vi "Get Active Row.vi"(8 "error in (no error)":errorcluster, 11 "Loop Data":T1) -> (0 "error out":errorcluster, 3 "Loop Data out":T1)   [LabVIEW 2016, in "System Mapping Tool.lvlib"]
uses:
  System Mapping Tool.lvlib
  TypeDefs/Loop Data.ctl
  TypeDefs/UI Refs.ctl
  NationalInstruments.VeriStand.SystemDefinitionAPI
  NationalInstruments.VeriStand.SystemStorageUI
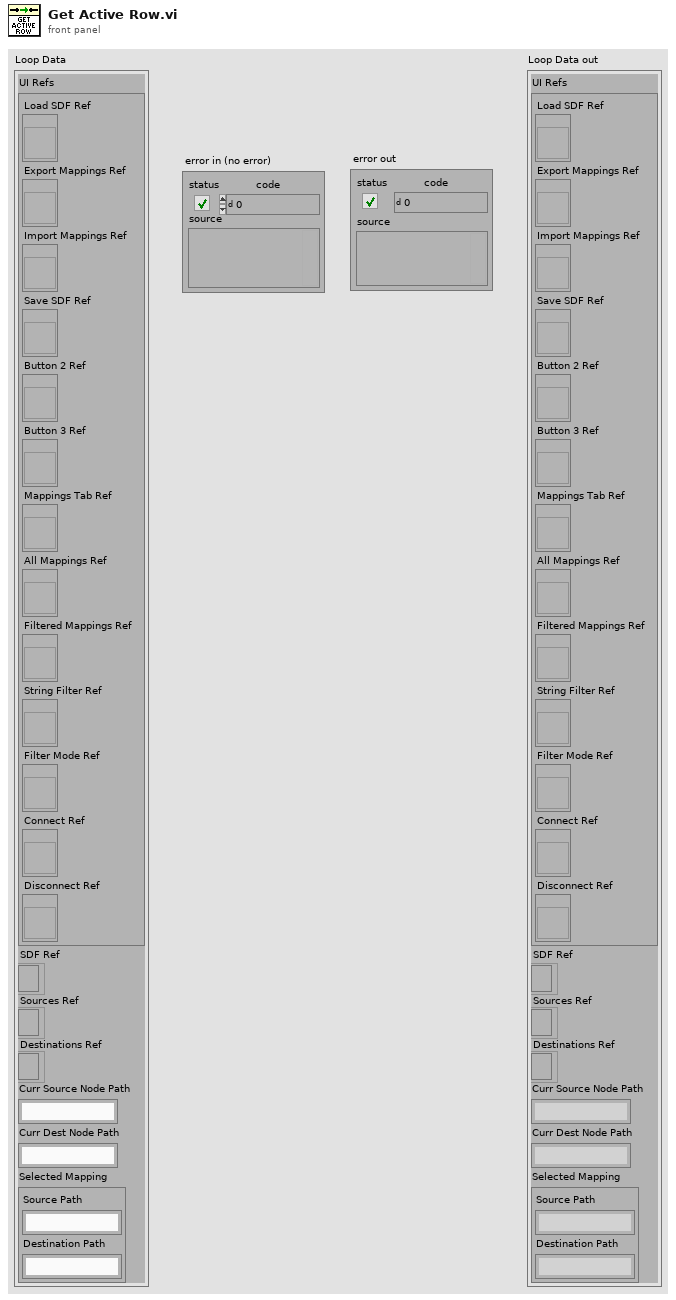
[diagram p1: front panel]
types:
  T1 = typedef "System Mapping Tool.lvlib/Loop Data.ctl" = cluster{"UI Refs":T2, "SDF Ref":refnum<k24>, "Sources Ref":refnum<k24>, "Destinations Ref":refnum<k24>, "Curr Source Node Path":string, "Curr Dest Node Path":string, "Selected Mapping":cluster{"Source Path":string, "Destination Path":string}}
  T2 = typedef "System Mapping Tool.lvlib/UI Refs.ctl" = cluster{"Load SDF Ref":refnum<vi>, "Export Mappings Ref":refnum<vi>, "Import Mappings Ref":refnum<vi>, "Save SDF Ref":refnum<vi>, "Button 2 Ref":refnum<vi>, "Button 3 Ref":refnum<vi>, "Mappings Tab Ref":refnum<vi>, "All Mappings Ref":refnum<vi>, "Filtered Mappings Ref":refnum<vi>, "String Filter Ref":refnum<vi>, "Filter Mode Ref":refnum<vi>, "Connect Ref":refnum<vi>, "Disconnect Ref":refnum<vi>}
  T3 = enum32{"All System Mappings", "Filtered Mappings by Node"}
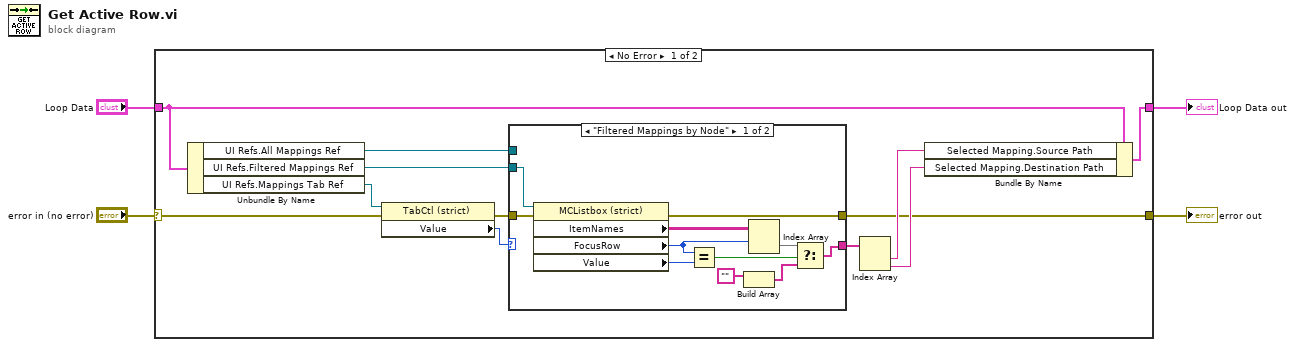
[diagram p0: block diagram]
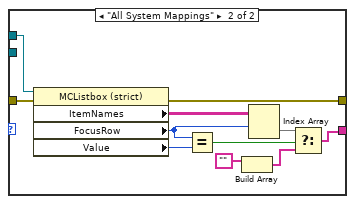
[diagram p2: hidden frame]
diagram:
  n1 = case shown="No Error" "error in (no error)" {
    selector: "error in (no error)" -> [w14 w40]
    tunnel: [w5 w40] -> w3
    tunnel: "Loop Data" -> [w16 w39]
    tunnel: [w15 w39] -> w1
    frame No Error {
      n2 = Unbundle By Name(w16) -> ("UI Refs.All Mappings Ref"=w9:refnum<vi>, "UI Refs.Filtered Mappings Ref"=w10:refnum<vi>, "UI Refs.Mappings Tab Ref"=w13:refnum<vi>)
      n3 = property class="TabCtl (strict)"(reference=w13, error in=w14) -> (error out=w11:errorcluster, "Value"=w12:T3)  [unwired: 1 out]
      n4 = case shown="\"Filtered Mappings by Node\"" w12 {
        tunnel: w11 -> [w27 w38]
        tunnel: w10 -> [w26 _]
        tunnel: w9 -> [_ w35]
        tunnel: [w24 w36] -> w5
        tunnel: [w19 w32] -> w8
        frame "Filtered Mappings by Node" {
          w22 = ""
          n5 = property class="MCListbox (strict)"(reference=w26, error in=w27) -> (error out=w24:errorcluster, "ItemNames"=w25:string[][], "FocusRow"=w17:i32, "Value"=w18:i32)  [unwired: 1 out]
          n6 = Equal?(x=w17, y=w18) -> (x = y?=w21:bool)
          n7 = Build Array(w22, w22) -> (w23:string[])
          n8 = Index Array(array=w25, index (row)=w17) -> (element=w20:string[])  [unwired: 1 in]
          n9 = Select(t=w20, s=w21, f=w23) -> (s? t:f=w19:string[])
        }
        frame "All System Mappings" {
          w29 = ""
          n10 = property class="MCListbox (strict)"(reference=w35, error in=w38) -> (error out=w36:errorcluster, "ItemNames"=w37:string[][], "FocusRow"=w33:i32, "Value"=w34:i32)  [unwired: 1 out]
          n11 = Equal?(x=w33, y=w34) -> (x = y?=w30:bool)
          n12 = Build Array(w29, w29) -> (w28:string[])
          n13 = Index Array(array=w37, index (row)=w33) -> (element=w31:string[])  [unwired: 1 in]
          n14 = Select(t=w31, s=w30, f=w28) -> (s? t:f=w32:string[])
        }
      }
      n15 = Index Array(array=w8) -> (element #1=w6:string, element #2=w7:string)  [unwired: 2 in]
      n16 = Bundle By Name(cluster=w16, "Selected Mapping.Source Path"=w6, "Selected Mapping.Destination Path"=w7) -> (w15:T1)
    }
    frame Error {
    }
  }
  "error out" <- w3
  "Loop Data out" <- w1
